vi "Uninit.vi"(2 "Container State":T1, 3 "Display State":T2) -> ()   [LabVIEW 2010, in "Twinkle Button.xctl"]
doc: "本VI是为《我和LabVIEW》一书编写的示例。\n关于本书的介绍请参考网页：\nhttp://ruanqizhen.spaces.live.com/blog/cns!5852D4F797C53FB6!4310.entry"
uses:
  Twinkle Button.xctl
  State.ctl
  C:/Program Files/National Instruments/LabVIEW 2010/resource/importtools/Common/Event/NISAST Event.lvclass
  <vilib>/_xctls/Container State.ctl
  <vilib>/_xctls/XControlSupport.lvlib
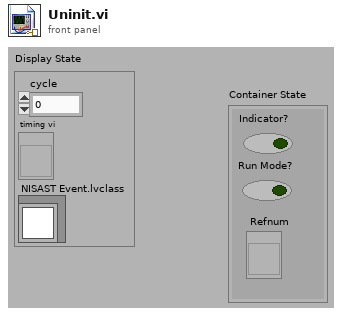
[diagram p1: front panel]
types:
  T1 = typedef "XControlSupport.lvlib/Container State.ctl" = cluster{"Indicator?":bool, "Run Mode?":bool, " Refnum":refnum<vi>}
  T2 = typedef "Twinkle Button.xctl/State.ctl" = cluster{"cycle":dbl, "timing vi":refnum<vi>, "NISAST Event.lvclass":refnum<class "NISAST Event.lvclass">}
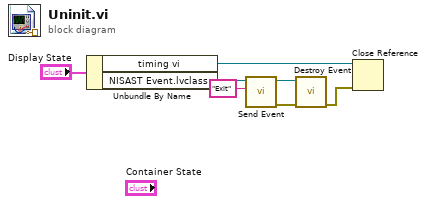
[diagram p0: block diagram]
diagram:
  n1 = Unbundle By Name("Display State") -> ("timing vi"=w2:refnum<vi>, "NISAST Event.lvclass"=w6:refnum<class "NISAST Event.lvclass">)
  n2 = call-dynamic "Send Event.vi"("Event Name"="Exit", "Event in"=w6) -> ("error out"=w3:errorcluster, "Event out"=w5:refnum<class "NISAST Event.lvclass">)  [unwired: 2 in, 6 out]
  n3 = call-dynamic "Destroy Event.vi"("error in (no error)"=w3, "Event in"=w5) -> ("error out"=w1:errorcluster)  [unwired: 9 out]
  n4 = Close Reference(reference=w2, error in (no error)=w1) -> ()  [unwired: 1 out]
